vi "TIFF-Open Stack.vi"(0 "stack in":T1={"file"=refnum, "IFD"=[], "offset"=0, "byte order"=enum."little-endian", "image size"=0, "IFD size"=0, "max frames"=0, "frames"=0}, 5 "file path (use dialog)":path, 11 "error in":errorcluster) -> (4 "stack out":T1={"file"=refnum, "IFD"=[], "offset"=0, "byte order"=enum."little-endian", "image size"=0, "IFD size"=0, "max frames"=0, "frames"=0}, 15 "error out":errorcluster)   [LabVIEW 2020]
uses:
  TIFF-Write State.ctl
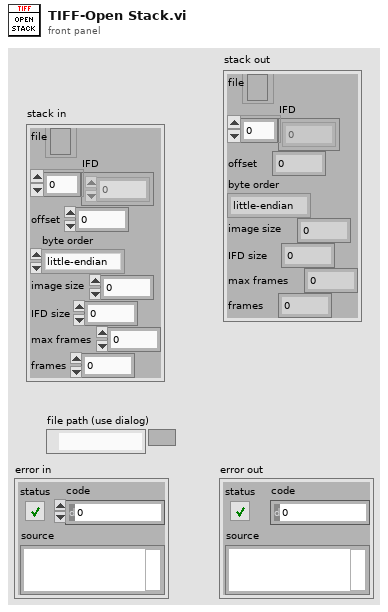
[diagram p1: front panel]
types:
  T1 = typedef "TIFF-Write State.ctl" = cluster{"file":refnum<file>, "IFD":u8[], "offset":u32, "byte order":enum16{"big-endian, network order", "native, host order", "little-endian"}, "image size":u32, "IFD size":u32, "max frames":u32, "frames":u32}
  T2 = enum16{"open", "replace", "create", "open or create", "replace or create", "replace or create with confirmation"}
  T3 = enum16{"big-endian, network order", "native, host order", "little-endian"}
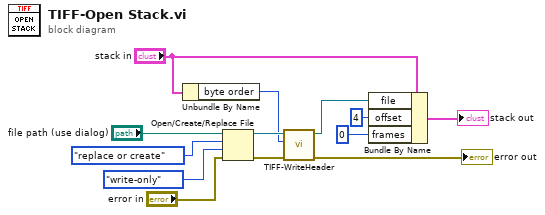
[diagram p0: block diagram]
diagram:
  n1 = Unbundle By Name("stack in") -> ("byte order"=w7:T3)
  n2 = Open/Create/Replace File(file path (use dialog)="file path (use dialog)", error in="error in", operation (0:open)=T2."replace or create", access (0:read/write)=enum16{"read/write", "read-only", "write-only"}."write-only") -> (refnum out=w11:refnum<file>, error out=w10:errorcluster)  [unwired: 2 in, 1 out]
  n3 = call "TIFF-WriteHeader.vi"("error in"=w10, "[IN] byte order"=w7, "[IN] refnum"=w11) -> ("error out"=→"error out":errorcluster, "[OUT] refnum"=w5:refnum<file>)  [unwired: 7 in]
  n4 = Bundle By Name(cluster="stack in", "file"=w5, "offset"=u32 4, "frames"=u32 0) -> (→"stack out":T1)
